vi "User.Timer.vi"(8 "error in (no error)":errorcluster, 10 "init (F)":bool, 11 "TIME [s]":dbl=3.0 format="%.2f") -> (0 "error out":errorcluster, 2 "trigger":bool, 3 "time elapsed [s]":dbl=3.0 format="%.2f")   [LabVIEW 2013]
doc: "CIT_TIMER \n(c) 1997 CIT\n-------------------\nV1.0\n\nTimer functie voor 'trage' processen (typisch >250ms).\n\nGenereert een stijgende flank op TRIGGER na het verstrijken van x-seconden (na init)? VI oproepen vanuit een While-LOOP met voldoende resolutie !\nReset timer en trigger met init=T\n\nAUTO_INIT: Als de knop 'auto_init' op false staat veranderdt er niets, in het andere geval geeft hij terug een init na het trigeren, zodat bij een aanroep vlak nadat er éénmaal getriggerd werd, de trigger puls terug uit is, tenzij de TIME voor een tweede keer verstreken is.\n\nBELANGRIJK : als dit VI niet minstens één keer per TIME wordt aangeroepen zal hij onthouden hoeveel trigerpulsen hij gemist heeft en deze pulsen zullen later (bij herhaaldelijk heraanroepen) gegeven worden. Hierdoor is het te meten object niet meer equidistant (in tijd), maar het aantal klopt wel\n\nINLOPEND:Indien u toch niet wenst dat de triger zichzelf inhaalt bij onvoldoende aanroepen, zet je inlopen op false."
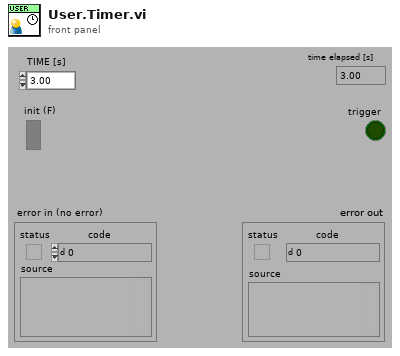
[diagram p1: front panel]
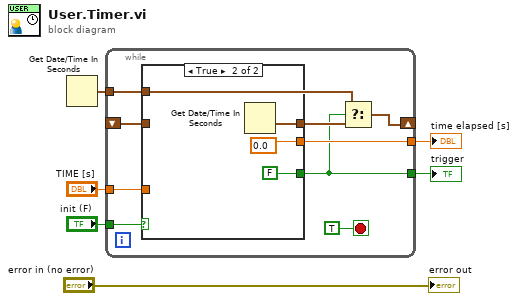
[diagram p0: block diagram]
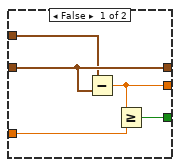
[diagram p2: hidden frame]
diagram:
  n1 = Get Date/Time In Seconds() -> (seconds since 1Jan1904=w3:timestamp)
  n2 = while {
    shift-right: [w8] -> _
    shift-left: _ -> [w15]
    tunnel: "TIME [s]" -> [w13]
    tunnel: "init (F)" -> [w12]
    tunnel: [w11] -> w4
    tunnel: w3 -> [w9]
    tunnel: [w7] -> w2
    stop <- TRUE stop-if-true
    n3 = case shown="True" w12 {
      tunnel: [w20 w23] -> w10
      tunnel: w15 -> [w20 _]
      tunnel: [w19 FALSE] -> w7
      tunnel: [w18 0.0] -> w11
      tunnel: w13 -> [w17 _]
      tunnel: w9 -> [w16 _]
      frame False {
        n4 = Subtract(x=w16, y=w20) -> (x-y=w18:dbl)
        n5 = Greater Or Equal?(x=w18, y=w17) -> (x >= y?=w19:bool)
      }
      frame True {
        n6 = Get Date/Time In Seconds() -> (seconds since 1Jan1904=w23:timestamp)
      }
    }
    n7 = Select(t=w9, s=w7, f=w10) -> (s? t:f=w8:timestamp)
  }
  "time elapsed [s]" <- w4
  "trigger" <- w2
  "error out" <- "error in (no error)"
